vi "2017-02-06 FullScan.vi"() -> ()   [LabVIEW 2016]
uses:
  <vilib>/Utility/error.llb/DialogType.ctl
  <vilib>/DAQmx/write.llb/DAQmx Write (Analog 1D DBL NChan 1Samp).vi
  <vilib>/DAQmx/write.llb/DAQmx Write (Analog DBL 1Chan 1Samp).vi
  <vilib>/DAQmx/create/channels.llb/DAQmx Create Channel (AO-Voltage-Basic).vi
  <vilib>/DAQmx/miscellaneous.llb/DAQmx Fill In Error Info.vi
panel:
  in  "Max Voltage 4":dbl=10.0
  in  "Min Voltage 2":dbl=-10.0
  in  "Stop 2":bool
  in  "Output Voltage 2":dbl[](array[numeric])
  in  "Physical Channel(s)  2":tag="Dev1/ao0"
  in  "Max Voltage 3":dbl=10.0
  in  "Min Voltage":dbl=-10.0
  in  "Stop":bool
  in  "Output Voltage":dbl[](array[numeric])
  in  "Physical Channel(s)":tag="Dev1/ao0"
  in  "Hold/Scan":enum32{"Hold", "Radio Selection 2"}(radio)
  in  "Voltage Step 2":dbl=0.1
  out "Current Voltage 2":dbl
  out "Next Voltage 2":dbl
  in  "Wait Time (ms) 2":dbl=100.0
  in  "Scan in X: Set to ao1\nScan in Y: Set to ao0":tag="Dev1/ao0"
  in  "Min Voltage Voltage 2":dbl=-10.0
  in  "Max Voltage 2":dbl=10.0
  in  "Voltage Step":dbl=0.1
  out "Current Voltage":dbl
  out "Next Voltage":dbl
  in  "Wait Time (ms)":dbl=100.0
  in  "Set this opposite to one above":tag="Dev1/ao0"
  in  "Min Voltage Voltage":dbl=-10.0
  in  "Max Voltage":dbl=10.0
  # "Use this stop button (for now)"
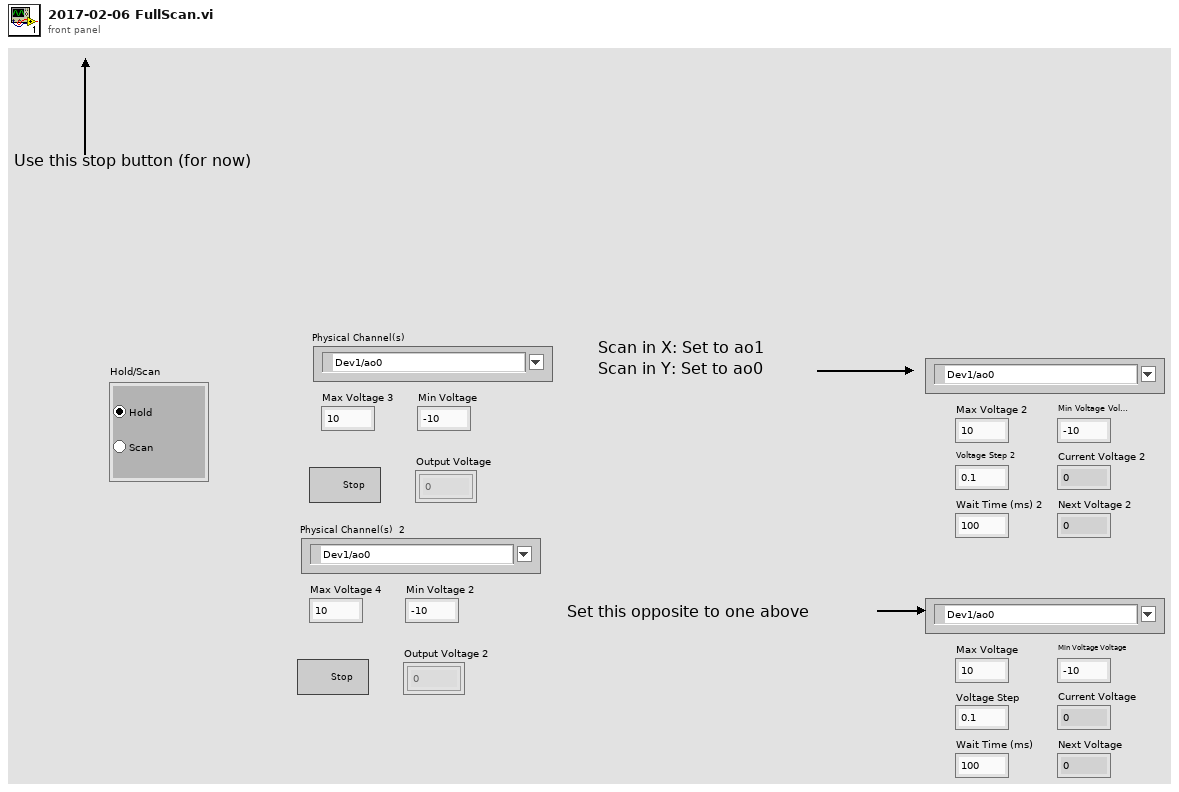
[diagram p1: front panel]
types:
  T1 = typedef "DialogType.ctl" = u16
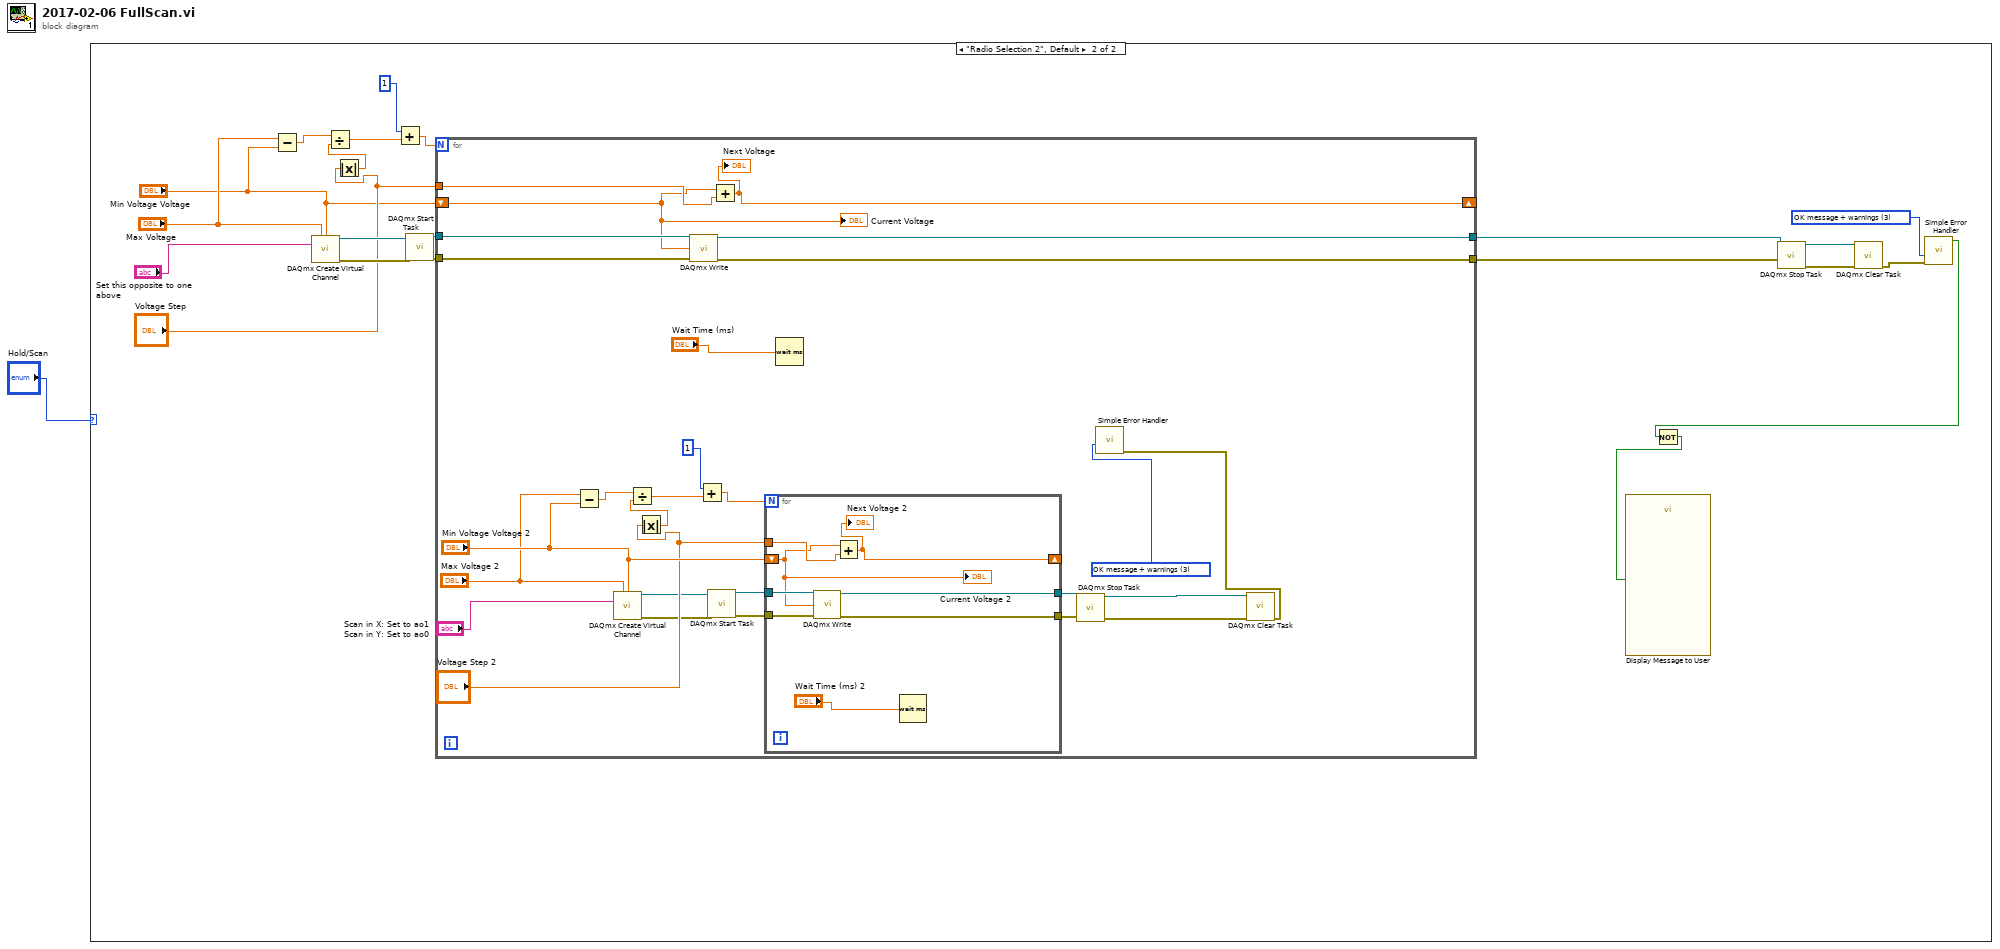
[diagram p0: block diagram]
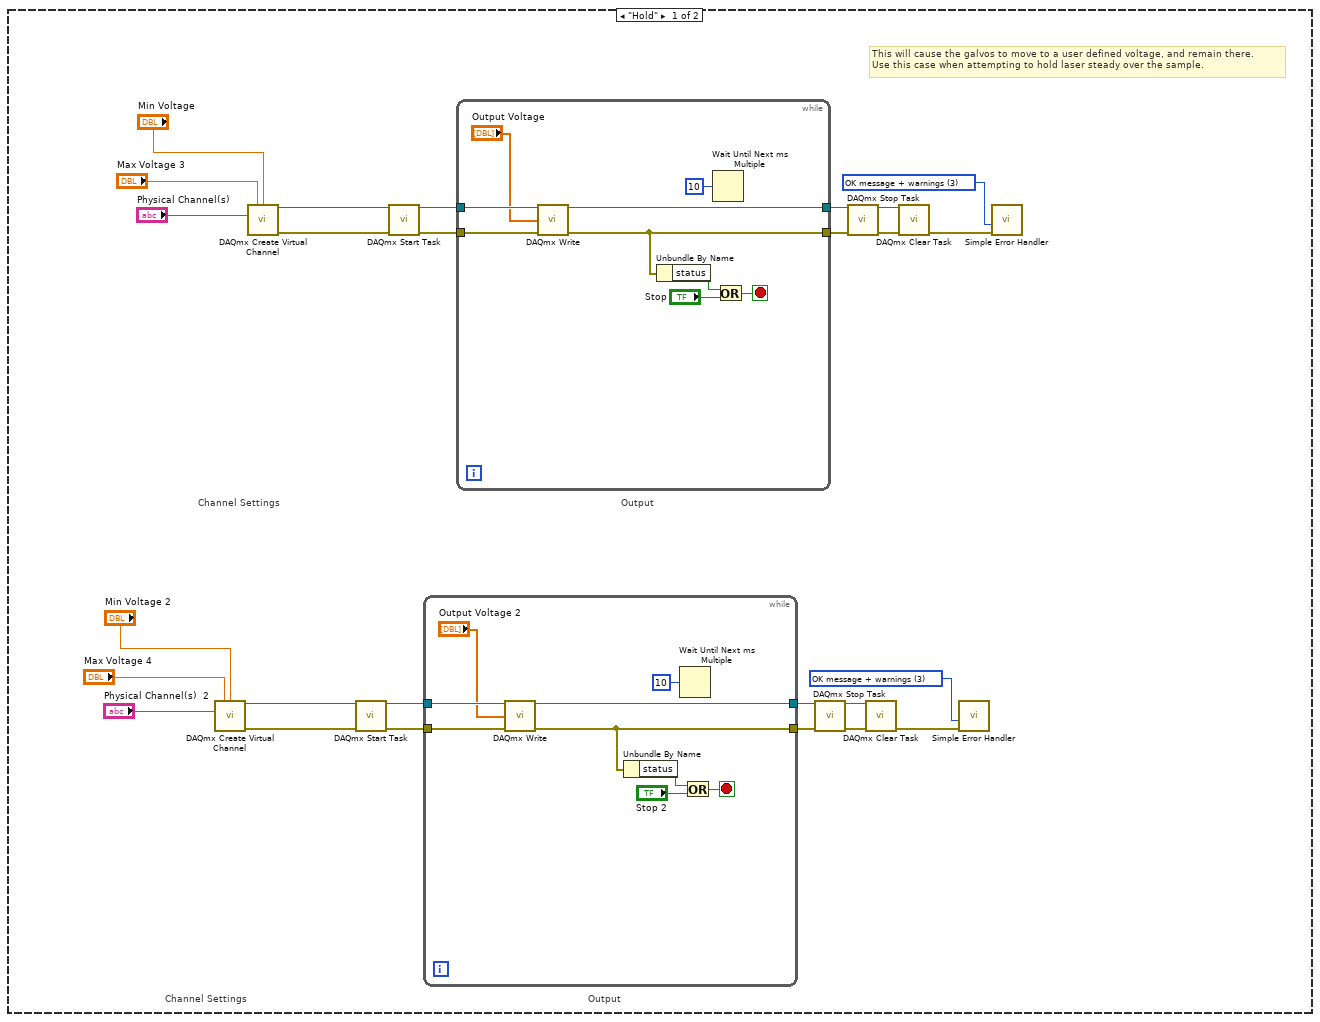
[diagram p2: hidden frame]
diagram:
  n1 = case shown="\"Radio Selection 2\", Default" "Hold/Scan" {
    frame "Hold" {
      w4 = T1 3 items=["no dialog", "OK message", "continue or stop message", "OK message + warnings", "continue/stop + warnings"] ("type of dialog (OK msg:1)")
      w17 = T1 3 items=["no dialog", "OK message", "continue or stop message", "OK message + warnings", "continue/stop + warnings"] ("type of dialog (OK msg:1)")
      # "Output"
      # "Channel Settings"
      # "This will cause the galvos to move to a user defined voltage, and remain there.\nUse this case when attempting to hold laser steady over the sample."
      # "Output"
      # "Channel Settings"
      n2 = call-poly <vilib>:"DAQmx Create Virtual Channel.vi"("maximum value"="Max Voltage 4", "minimum value"="Min Voltage 2", "physical channels"="Physical Channel(s)  2") -> ("task out"=w12:refnum<k21>, "error out"=w11:errorcluster)  [unwired: 11 in]
      n3 = call-poly <vilib>:"DAQmx Create Virtual Channel.vi"("maximum value"="Max Voltage 3", "minimum value"="Min Voltage", "physical channels"="Physical Channel(s)") -> ("task out"=w25:refnum<k21>, "error out"=w24:errorcluster)  [unwired: 11 in]
      n4 = call <vilib>:"DAQmx Start Task.vi"("task/channels in"=w12, "error in"=w11) -> ("task out"=w10:refnum<k21>, "error out"=w9:errorcluster)  [unwired: 12 in]
      n5 = call <vilib>:"DAQmx Start Task.vi"("task/channels in"=w25, "error in"=w24) -> ("task out"=w23:refnum<k21>, "error out"=w22:errorcluster)  [unwired: 12 in]
      n6 = while {
        tunnel: w10 -> [w36]
        tunnel: w9 -> [w35]
        tunnel: [w30] -> w7
        tunnel: [w34] -> w8
        stop <- w28 stop-if-true
        n7 = call-poly <vilib>:"DAQmx Write.vi"("task/channels in"=w36, "data"="Output Voltage 2", "error in"=w35) -> ("task out"=w34:refnum<k21>, "error out"=w30:errorcluster)  [unwired: 10 in, 1 out]
        n8 = Unbundle By Name(w30) -> ("status"=w32:bool)
        n9 = Wait Until Next ms Multiple(millisecond multiple=u32 10) -> ()  [unwired: 1 out]
        n10 = Or(x=w32, y="Stop 2") -> (x .or. y?=w28:bool)
      }
      n11 = while {
        tunnel: w23 -> [w45]
        tunnel: w22 -> [w44]
        tunnel: [w39] -> w20
        tunnel: [w43] -> w21
        stop <- w37 stop-if-true
        n12 = call-poly <vilib>:"DAQmx Write.vi"("task/channels in"=w45, "data"="Output Voltage", "error in"=w44) -> ("task out"=w43:refnum<k21>, "error out"=w39:errorcluster)  [unwired: 10 in, 1 out]
        n13 = Unbundle By Name(w39) -> ("status"=w41:bool)
        n14 = Wait Until Next ms Multiple(millisecond multiple=u32 10) -> ()  [unwired: 1 out]
        n15 = Or(x=w41, y="Stop") -> (x .or. y?=w37:bool)
      }
      n16 = call <vilib>:"DAQmx Stop Task.vi"("task/channels in"=w8, "error in"=w7) -> ("task out"=w6:refnum<k21>, "error out"=w5:errorcluster)  [unwired: 12 in]
      n17 = call <vilib>:"DAQmx Stop Task.vi"("task/channels in"=w21, "error in"=w20) -> ("task out"=w19:refnum<k21>, "error out"=w18:errorcluster)  [unwired: 12 in]
      n18 = call <vilib>:"DAQmx Clear Task.vi"("task in"=w6, "error in"=w5) -> ("error out"=w14:errorcluster)  [unwired: 13 in]
      n19 = call <vilib>:"DAQmx Clear Task.vi"("task in"=w19, "error in"=w18) -> ("error out"=w27:errorcluster)  [unwired: 13 in]
      n20 = call <vilib>:"Simple Error Handler.vi"("type of dialog (OK msg:1)"=w4, "error in (no error)"=w14) -> ()  [unwired: 3 in, 5 out]
      n21 = call <vilib>:"Simple Error Handler.vi"("type of dialog (OK msg:1)"=w17, "error in (no error)"=w27) -> ()  [unwired: 3 in, 5 out]
    }
    frame "Radio Selection 2", Default {
      w57 = T1 3 items=["no dialog", "OK message", "continue or stop message", "OK message + warnings", "continue/stop + warnings"] ("type of dialog (OK msg:1)")
      n22 = Subtract(x="Max Voltage", y="Min Voltage Voltage") -> (x-y=w54:dbl)
      n23 = call-poly <vilib>:"DAQmx Create Virtual Channel.vi"("maximum value"="Max Voltage", "minimum value"="Min Voltage Voltage", "physical channels"="Set this opposite to one above") -> ("task out"=w65:refnum<k21>, "error out"=w64:errorcluster)  [unwired: 11 in]
      n24 = Absolute Value(x="Voltage Step") -> (abs(x)=w52:dbl)
      n25 = Divide(x=w54, y=w52) -> (x/y=w50:dbl)
      n26 = Add(x=1, y=w50) -> (x+y=w48:dbl)
      n27 = call <vilib>:"DAQmx Start Task.vi"("task/channels in"=w65, "error in"=w64) -> ("task out"=w63:refnum<k21>, "error out"=w62:errorcluster)  [unwired: 12 in]
      n28 = for {
        N: w48 -> [_]
        tunnel: w63 -> [w93]
        tunnel: w62 -> [w92]
        tunnel: [w91] -> w61
        tunnel: [w89] -> w60
        tunnel: "Voltage Step" -> [w90]
        shift-right: [w87] -> _
        shift-left: "Min Voltage Voltage" -> [w88]
        w77 = T1 3 items=["no dialog", "OK message", "continue or stop message", "OK message + warnings", "continue/stop + warnings"] ("type of dialog (OK msg:1)")
        n29 = Subtract(x="Max Voltage 2", y="Min Voltage Voltage 2") -> (x-y=w80:dbl)
        n30 = call-poly <vilib>:"DAQmx Create Virtual Channel.vi"("maximum value"="Max Voltage 2", "minimum value"="Min Voltage Voltage 2", "physical channels"="Scan in X: Set to ao1\nScan in Y: Set to ao0") -> ("task out"=w69:refnum<k21>, "error out"=w70:errorcluster)  [unwired: 11 in]
        n31 = Absolute Value(x="Voltage Step 2") -> (abs(x)=w82:dbl)
        n32 = Divide(x=w80, y=w82) -> (x/y=w84:dbl)
        n33 = call-poly <vilib>:"DAQmx Write.vi"("task/channels in"=w93, "data"=w88, "error in"=w92) -> ("task out"=w89:refnum<k21>, "error out"=w91:errorcluster)  [unwired: 10 in, 1 out]
        n34 = Add(x=1, y=w84) -> (x+y=w85:dbl)
        n35 = call <vilib>:"DAQmx Start Task.vi"("task/channels in"=w69, "error in"=w70) -> ("task out"=w71:refnum<k21>, "error out"=w72:errorcluster)  [unwired: 12 in]
        n36 = Add(x=w88, y=w90) -> (x+y=w87:dbl)
        "Next Voltage" <- w87
        n37 = for {
          N: w85 -> [_]
          tunnel: w71 -> [w101]
          tunnel: w72 -> [w100]
          tunnel: [w99] -> w73
          tunnel: [w97] -> w74
          tunnel: "Voltage Step 2" -> [w98]
          shift-right: [w95] -> _
          shift-left: "Min Voltage Voltage 2" -> [w96]
          n38 = call-poly <vilib>:"DAQmx Write.vi"("task/channels in"=w101, "data"=w96, "error in"=w100) -> ("task out"=w97:refnum<k21>, "error out"=w99:errorcluster)  [unwired: 10 in, 1 out]
          n39 = Add(x=w96, y=w98) -> (x+y=w95:dbl)
          "Next Voltage 2" <- w95
          n40 = Wait (ms)(milliseconds to wait="Wait Time (ms) 2") -> ()  [unwired: 1 out]
          "Current Voltage 2" <- w96
        }
        n41 = Wait (ms)(milliseconds to wait="Wait Time (ms)") -> ()  [unwired: 1 out]
        n42 = call <vilib>:"DAQmx Stop Task.vi"("task/channels in"=w74, "error in"=w73) -> ("task out"=w76:refnum<k21>, "error out"=w75:errorcluster)  [unwired: 12 in]
        n43 = call <vilib>:"DAQmx Clear Task.vi"("task in"=w76, "error in"=w75) -> ("error out"=w78:errorcluster)  [unwired: 13 in]
        n44 = call <vilib>:"Simple Error Handler.vi"("type of dialog (OK msg:1)"=w77, "error in (no error)"=w78) -> ()  [unwired: 3 in, 5 out]
        "Current Voltage" <- w88
      }
      n45 = call <vilib>:"DAQmx Stop Task.vi"("task/channels in"=w60, "error in"=w61) -> ("task out"=w58:refnum<k21>, "error out"=w59:errorcluster)  [unwired: 12 in]
      n46 = call <vilib>:"DAQmx Clear Task.vi"("task in"=w58, "error in"=w59) -> ("error out"=w56:errorcluster)  [unwired: 13 in]
      n47 = call <vilib>:"Simple Error Handler.vi"("type of dialog (OK msg:1)"=w57, "error in (no error)"=w56) -> ("error?"=w47:bool)  [unwired: 3 in, 4 out]
      n48 = Not(x=w47) -> (.not. x?=w46:bool)
      n49 = call "Display Message to User"("Enable"=w46) -> ()  [unwired: 9 in, 2 out]
    }
  }
